vi "Weather.vi"() -> ()   [LabVIEW 2015]
uses:
  <vilib>/httpClient/LabVIEWHTTPClient.lvlib
panel:
  out "Humidity(%)":i32
  out "Temperature":dbl(slide) scale=0.0..50.0
  out "Humidity":i32(slide) scale=0.0..100.0
  out "Pressure":i32(knob) scale=0.0..1500.0
  out "Wind Speed":dbl(slide) scale=0.0..35.0
  out "Wind Speed (m/sec)":string
  out "Pressure (mm)":string
  out "Temperature (C)":string
  out "Conditions":string
  out "body":string
  out "headers":string
  in  "stop":bool
  in  "City":string
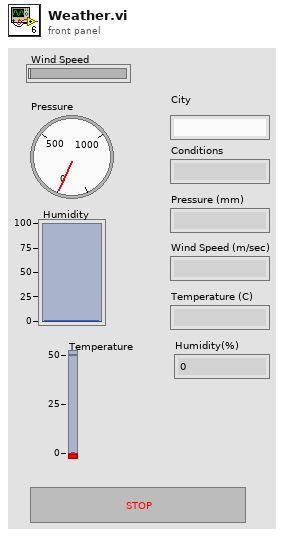
[diagram p1: front panel]
types:
  T1 = enum16{"open", "replace", "create", "open or create", "replace or create", "replace or create with confirmation"}
  T2 = typedef "LabVIEWHTTPClient.lvlib/ClientHandle.ctl" = refnum<k1>
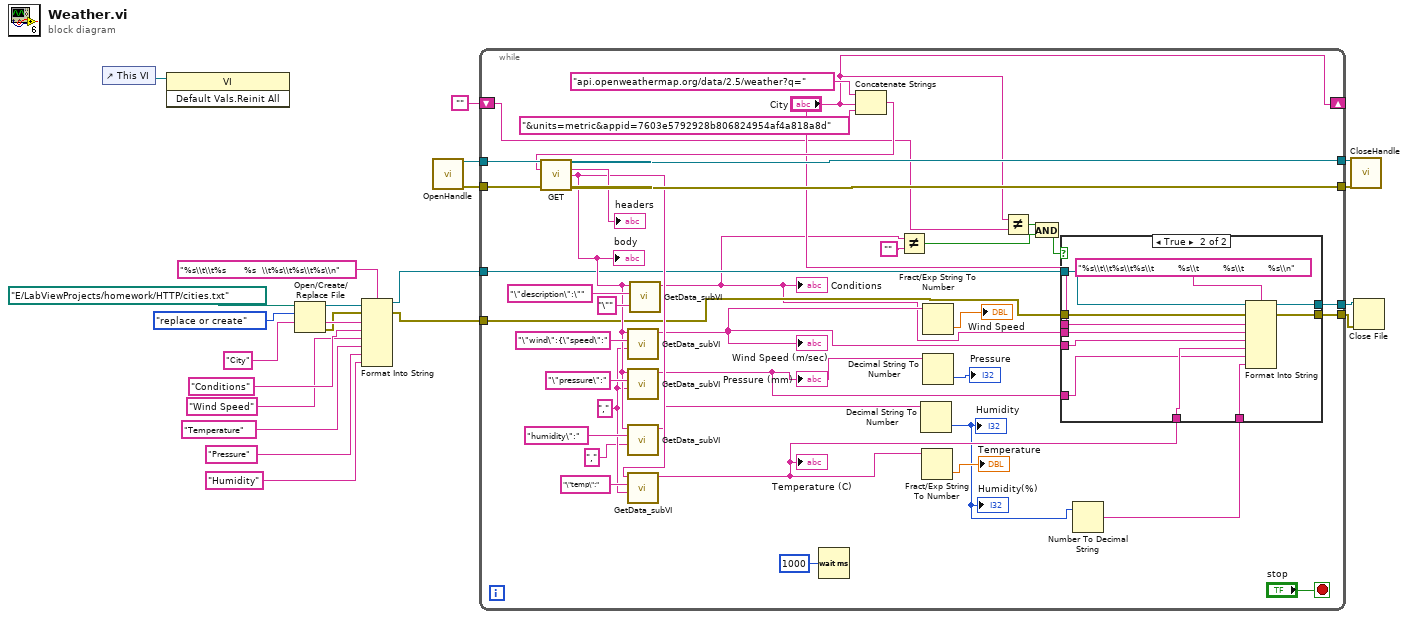
[diagram p0: block diagram]
diagram:
  n1 = control-ref of="This VI"() -> (w17:refnum<vi>)
  n2 = invoke class="VI" method="Default Vals.Reinit All"(reference=w17) -> ()  [unwired: 2 in, 3 out]
  n3 = Open/Create/Replace File(file path (use dialog)=path "E:/LabViewProjects/homework/HTTP/cities.txt", operation (0:open)=T1."replace or create") -> (refnum out=w8:refnum<file>, error out=w7:errorcluster)  [unwired: 4 in, 1 out]
  n4 = Format Into String ("Format Into File")(format string="%s\\t\\t%s      %s  \\t%s\\t%s\\t%s\\n", initial string=w8, error in=w7, "City" ("input 1"), "Conditions" ("input 1"), "Wind Speed" ("input 1"), "Temperature" ("input 1"), "Pressure" ("input 1"), "Humidity" ("input 1")) -> (resulting string=w4:refnum<file>, error out=w3:errorcluster)
  n5 = call <vilib>:"OpenHandle.vi"() -> ("client handle out"=w21:T2, "error out"=w20:errorcluster)  [unwired: 14 in]
  n6 = while {
    tunnel: w21 -> [w60]
    tunnel: w20 -> [w59]
    tunnel: [w52] -> w19
    tunnel: [w51] -> w18
    tunnel: [w39] -> w6
    tunnel: [w38] -> w5
    tunnel: w4 -> [w37]
    tunnel: w3 -> [w36]
    shift-right: ["City"] -> _
    shift-left: "" -> [w29]
    stop <- "stop" stop-if-true
    w43 = "," ("word after")
    n7 = Wait (ms)(milliseconds to wait=u32 1000) -> ()  [unwired: 1 out]
    n8 = Concatenate Strings("api.openweathermap.org/data/2.5/weather?q=" ("url"), "City", "&units=metric&appid=7603e5792928b806824954af4a818a8d" ("url")) -> (w54:string)
    n9 = call <vilib>:"GET.vi"("client handle"=w60, "url"=w54, "error in (no error)"=w59) -> ("client handle out"=w52:T2, "headers"=→"headers":string, "body"=w45:string, "error out"=w51:errorcluster)  [unwired: 9 in]
    "body" <- w45
    n10 = call "GetData_subVI.vi"("word after"=w43, "word before"="\"wind\":{\"speed\":", "body in"=w45) -> ("data out"=w35:string)  [unwired: 8 in]
    "Wind Speed (m/sec)" <- w35
    n11 = call "GetData_subVI.vi"("word after"=w43, "word before"="\"pressure\":", "body in"=w45) -> ("data out"=w33:string)  [unwired: 8 in]
    "Pressure (mm)" <- w33
    n12 = call "GetData_subVI.vi"("word after"=",", "word before"="humidity\":", "body in"=w45) -> ("data out"=w32:string)  [unwired: 8 in]
    n13 = call "GetData_subVI.vi"("word after"=w43, "word before"="\"temp\":", "body in"=w45) -> ("data out"=w34:string)  [unwired: 8 in]
    "Temperature (C)" <- w34
    n14 = call "GetData_subVI.vi"("word after"="\"", "word before"="\"description\":\"", "body in"=w45) -> ("data out"=w27:string)  [unwired: 8 in]
    "Conditions" <- w27
    n15 = Not Equal?(x=w27, y="") -> (x != y?=w24:bool)
    n16 = Decimal String To Number(string=w32) -> (number=w23:i32)  [unwired: 2 in, 1 out]
    "Humidity" <- w23
    "Humidity(%)" <- w23
    n17 = Fract/Exp String To Number(string=w34) -> (number=→"Temperature":dbl)  [unwired: 3 in, 1 out]
    n18 = Fract/Exp String To Number(string=w35) -> (number=→"Wind Speed":dbl)  [unwired: 3 in, 1 out]
    n19 = Decimal String To Number(string=w33) -> (number=→"Pressure":i32)  [unwired: 2 in, 1 out]
    n20 = Not Equal?(x="City", y=w29) -> (x != y?=w26:bool)
    n21 = And(x=w26, y=w24) -> (x .and. y?=w25:bool)
    n22 = Number To Decimal String(number=w23) -> (decimal integer string=w22:string)  [unwired: 1 in]
    n23 = case shown="True" w25 {
      tunnel: [w62 w72] -> w39
      tunnel: [w61 w71] -> w38
      tunnel: w37 -> [w62 w70]
      tunnel: w36 -> [w61 w69]
      tunnel: "City" -> [_ w68]
      tunnel: w27 -> [_ w67]
      tunnel: w35 -> [_ w66]
      tunnel: w34 -> [_ w65]
      tunnel: w33 -> [_ w64]
      tunnel: w22 -> [_ w63]
      frame False {
      }
      frame True {
        n24 = Format Into String ("Format Into File")(format string="%s\\t\\t%s\\t%s\\t        %s\\t        %s\\t        %s\\n", initial string=w70, error in=w69, w68, w67, w66, w65, w64, w63) -> (resulting string=w72:refnum<file>, error out=w71:errorcluster)
      }
    }
  }
  n25 = call <vilib>:"CloseHandle.vi"("client handle"=w19, "error in (no error)"=w18) -> ()  [unwired: 13 in, 1 out]
  n26 = Close File(refnum=w6, error in=w5) -> ()  [unwired: 2 out]
